vi "S4GUI_002.vi"(7 "Tab ObsEng":enum32{"Obs", "CCD modes", "Eng"}(tab)) -> ()   [LabVIEW 2018] (continued)
          tunnel: w10386 -> [w10388 w10421]
          tunnel: w10385 -> [w10387 w10420]
          tunnel: [w10387 w10398] -> w10384
          tunnel: [w10388 w10399] -> w10383
          frame False {
          }
          frame True {
            # "Carrega a maior temperatura\nentre target atual e o target do controle."
            # "Carrega o valor da temperatura target de acordo com a conf CCD"
            n4383 = call-dynamic "Read AcquisitionD.vi"("error in (no error)"=w10420, "S4ACS_GUI in"=w10421) -> ("error out"=w10424:errorcluster, "Acquisition.lvclass"=w10425:refnum<class "Acquisition.lvclass">, "S4ACS_GUI out"=w10394:refnum<class "S4GUI.lvclass">)  [unwired: 7 in]
            n4384 = call-dynamic "Read Channel.vi"("error in (no error)"=w10424, "Acquisition in"=w10425) -> ("error out"=w10415:errorcluster, "Channel.lvclass"=w10416:refnum<class "Channel.lvclass">, "Acquisition out"=w10395:refnum<class "Acquisition.lvclass">)  [unwired: 7 in]
            n4385 = call-dynamic "ValidateConfig.vi"("error in (no error)"=w10415, "Channel in"=w10416) -> ("error out"=w10409:errorcluster, "Channel out"=w10410:refnum<class "Channel.lvclass">)  [unwired: 7 in, 1 out]
            n4386 = call-dynamic "Read Interface.vi"("error in (no error)"=w10409, "Channel in"=w10410) -> ("error out"=w10413:errorcluster, "Interface.lvclass"=w10414:refnum<class "Interface.lvclass">, "Channel out"=w10418:refnum<class "Channel.lvclass">)  [unwired: 7 in]
            n4387 = call-dynamic "Read Temperature.vi"("error in (no error)"=w10413, "Interface in"=w10414) -> ("error out"=w10412:errorcluster, "Temperature"=w10408:i8, "Interface out"=w10411:refnum<class "Interface.lvclass">)  [unwired: 7 in]
            n4388 = Greater?(x=w10408, y="Target Temp 4") -> (0:w10393:bool)
            n4389 = Select(t=w10408, s=w10393, f="Target Temp 4") -> (s? t:f=w10407:i32)
            n4390 = call-dynamic "Write Temperature.vi"("error in (no error)"=w10412, "Temperature"=w10407, "Interface in"=w10411) -> ("error out"=w10417:errorcluster, "Interface out"=w10419:refnum<class "Interface.lvclass">)  [unwired: 7 in]
            n4391 = call-dynamic "Write Interface.vi"("error in (no error)"=w10417, "Interface.lvclass"=w10419, "Channel in"=w10418) -> ("error out"=w10396:errorcluster, "Channel out"=w10397:refnum<class "Channel.lvclass">)  [unwired: 7 in]
            n4392 = case shown="True" w10393 {
              tunnel: w10396 -> [w10450 w10455]
              tunnel: w10397 -> [w10449 w10457]
              tunnel: [w10448 w10457] -> w10392
              tunnel: [w10447 w10460] -> w10389
              tunnel: w10394 -> [w10427 w10456]
              tunnel: [w10427 w10459] -> w10390
              tunnel: w10395 -> [w10426 w10452]
              tunnel: [w10426 w10458] -> w10391
              frame False {
                n4393 = call-dynamic "Read State Machine.vi"("error in (no error)"=w10450, "Device in"=w10449) -> ("error out"=w10429:errorcluster, "State Machine.lvclass"=w10436:refnum<class "State Machine.lvclass">, "Device out"=w10445:refnum<class "Channel.lvclass">)  [unwired: 7 in]
                n4394 = call-dynamic "Read ref StatesQueue.vi"("error in (no error)"=w10429, "State Machine in"=w10436) -> ("error out"=w10439:errorcluster, "ref StatesQueue"=w10433:refnum<queue>, "State Machine out"=w10435:refnum<class "State Machine.lvclass">)  [unwired: 7 in]
                n4395 = Flush Queue(queue=w10433, error in (no error)=w10439) -> (queue out=w10432:refnum<queue>, error out=w10441:errorcluster)  [unwired: 1 out]
                n4396 = Enqueue Element(queue=w10432, element=u32 35 ("State"), error in (no error)=w10441) -> (queue out=w10431:refnum<queue>, error out=w10442:errorcluster)  [unwired: 1 in, 1 out]
                n4397 = Enqueue Element(queue=w10431, element=u32 37 ("State"), error in (no error)=w10442) -> (queue out=w10430:refnum<queue>, error out=w10440:errorcluster)  [unwired: 1 in, 1 out]
                n4398 = call-dynamic "Write ref StatesQueue.vi"("error in (no error)"=w10440, "ref StatesQueue"=w10430, "State Machine in"=w10435) -> ("error out"=w10428:errorcluster, "State Machine out"=w10434:refnum<class "State Machine.lvclass">)  [unwired: 7 in]
                n4399 = call "Next State.vi"("error in (no error)"=w10428, "New_State"=u32 0, "State Machine in"=w10434) -> ("error out"=w10446:errorcluster, "State Machine out"=w10444:refnum<class "State Machine.lvclass">)  [unwired: 7 in]
                n4400 = call-dynamic "Write State Machine.vi"("error in (no error)"=w10446, "State Machine.lvclass"=w10444, "Device in"=w10445) -> ("error out"=w10447:errorcluster, "Device out"=w10448:refnum<class "Channel.lvclass">)  [unwired: 7 in]
              }
              frame True {
                # "input error"
                n4401 = call-dynamic "Read SET temp error mode.vi"("error in (no error)"=w10455, "S4GUI in"=w10456) -> ("error out"=w10454:errorcluster, "SET temp error mode"=w10451:bool, "S4GUI out"=w10453:refnum<class "S4GUI.lvclass">)  [unwired: 7 in]
                n4402 = case shown="True" w10451 {
                  tunnel: [w10469 w10482] -> w10460
                  tunnel: [w10468 w10490] -> w10459
                  tunnel: [w10464 w10489] -> w10458
                  tunnel: w10454 -> [w10463 w10482]
                  tunnel: w10453 -> [w10461 w10490]
                  tunnel: w10452 -> [w10462 w10489]
                  frame False {
                    # "last error msg"
                    n4403 = call-dynamic "Read sync.vi"("error in (no error)"=w10463, "S4ACS_GUI in"=w10461) -> ("error out"=w10465:errorcluster, "sync"=w10466:bool, "S4ACS_GUI out"=w10467:refnum<class "S4GUI.lvclass">)  [unwired: 7 in]
                    n4404 = case shown="False" w10466 {
                      tunnel: w10465 -> [w10472 w10481]
                      tunnel: [w10471 w10480] -> w10469
                      tunnel: [w10475 w10479] -> w10468
                      tunnel: w10467 -> [w10475 w10477]
                      tunnel: w10462 -> [w10473 w10476]
                      tunnel: [w10470 w10476] -> w10464
                      frame False {
                        n4405 = call-dynamic "Write Acq_state.vi"("error in (no error)"=w10472, "Acq_state"=u32 240, "Acquisition in"=w10473) -> ("error out"=w10471:errorcluster, "Acquisition out"=w10470:refnum<class "Acquisition.lvclass">)  [unwired: 7 in]
                      }
                      frame True {
                        n4406 = call-dynamic "Write Obs_state.vi"("error in (no error)"=w10481, "Obs_state"=u32 240, "S4ACS_GUI in"=w10477) -> ("error out"=w10480:errorcluster, "S4ACS_GUI out"=w10479:refnum<class "S4GUI.lvclass">)  [unwired: 7 in]
                      }
                    }
                  }
                  frame True {
                    w10484 = FALSE ("Wait Until Done")
                    # "popup msg"
                    n4407 = call <vilib>:"Application Directory.vi"() -> ("Application Directory"=w10488:path)
                    n4408 = Build Path(base path=w10488, name or relative path="MsgSetTemp.vi") -> (appended path=w10485:path)
                    n4409 = Open VI Reference(vi path=w10485) -> (vi reference=w10486:refnum<vi>, error out=w10487:errorcluster)  [unwired: 5 in]
                    n4410 = invoke class="VI" method="Run VI"(reference=w10486, error in=w10487, "Wait until done"=w10484, "Auto Dispose Ref"=w10484) -> ()  [unwired: 1 in, 5 out]
                  }
                }
              }
            }
            n4411 = Number To Decimal String(number="Target Temp 4") -> (decimal integer string=w10406:string)  [unwired: 1 in]
            n4412 = call-dynamic "Write Channel.vi"("error in (no error)"=w10389, "Channel.lvclass"=w10392, "Acquisition in"=w10391) -> ("error out"=w10422:errorcluster, "Acquisition out"=w10423:refnum<class "Acquisition.lvclass">)  [unwired: 7 in]
            n4413 = Concatenate Strings("SET TEMP [" ("User Event"), w10406, "] CLICKED - CH4" ("User Event")) -> (w10405:string)
            n4414 = call-dynamic "Write AcquisitionD.vi"("error in (no error)"=w10422, "Acquisition.lvclass"=w10423, "S4ACS_GUI in"=w10390) -> ("error out"=w10400:errorcluster, "S4ACS_GUI out"=w10401:refnum<class "S4GUI.lvclass">)  [unwired: 7 in]
            n4415 = call-dynamic "Write User Event.vi"("error in (no error)"=w10400, "User Event"=w10405, "S4GUI in"=w10401) -> ("error out"=w10398:errorcluster, "S4GUI out"=w10399:refnum<class "S4GUI.lvclass">)  [unwired: 7 in]
          }
        }
      }
      event "SET Temp message": Value Change {
        # "Seleção do modo de apresentação da\nmensagem de erro para o SET de \ntemperatura manual:\nF: via Last Error em vermelho (S4GUI:HandleObservation.vi);\nT: via janela de popup (MsgTempPopup.vi)."
        n4416 = event-data() -> ("NewVal"=w10493:bool)  [unwired: 1 in]
        n4417 = call-dynamic "Write SET temp error mode.vi"("error in (no error)"=w10494, "SET temp error mode"=w10493, "S4GUI in"=w10495) -> ("error out"=w10491:errorcluster, "S4GUI out"=w10492:refnum<class "S4GUI.lvclass">)  [unwired: 7 in]
      }
      event "Avança Estado": Value Change {
        n4418 = event-data() -> ()  [unwired: 1 in, 4 out]
        n4419 = call-dynamic "Read Sync Box.lvclass.vi"("error in (no error)"=w10504, "SPARC4_AC in"=w10505) -> ("error out"=w10517:errorcluster, "Sync Box.lvclass"=w10518:refnum<class "Sync Box.lvclass">, "SPARC4_AC out"=w10509:refnum<class "S4GUI.lvclass">)  [unwired: 7 in]
        n4420 = call-dynamic "Read Trigger.lvclass.vi"("error in (no error)"=w10517, "Sync Box in"=w10518) -> ("error out"=w10515:errorcluster, "Trigger.lvclass"=w10516:refnum<class "Trigger.lvclass">, "Sync Box out"=w10512:refnum<class "Sync Box.lvclass">)  [unwired: 7 in]
        n4421 = call-dynamic "Read State Machine.vi"("error in (no error)"=w10515, "Device in"=w10516) -> ("error out"=w10501:errorcluster, "State Machine.lvclass"=w10502:refnum<class "State Machine.lvclass">, "Device out"=w10513:refnum<class "Trigger.lvclass">)  [unwired: 7 in]
        n4422 = call-dynamic "Read State.vi"("error in (no error)"=w10501, "State Machine in"=w10502) -> ("error out"=w10497:errorcluster, "State"=w10500:i32, "State Machine out"=w10498:refnum<class "State Machine.lvclass">)  [unwired: 7 in]
        n4423 = Increment(x=w10500) -> (x+1=w10499:i32)
        n4424 = call "Next State.vi"("error in (no error)"=w10497, "New_State"=w10499, "State Machine in"=w10498) -> ("error out"=w10511:errorcluster, "State Machine out"=w10514:refnum<class "State Machine.lvclass">)  [unwired: 7 in]
        n4425 = call-dynamic "Write State Machine.vi"("error in (no error)"=w10511, "State Machine.lvclass"=w10514, "Device in"=w10513) -> ("error out"=w10507:errorcluster, "Device out"=w10506:refnum<class "Trigger.lvclass">)  [unwired: 7 in]
        n4426 = call-dynamic "Write Trigger.lvclass.vi"("error in (no error)"=w10507, "Trigger.lvclass"=w10506, "Sync Box in"=w10512) -> ("error out"=w10508:errorcluster, "Sync Box out"=w10510:refnum<class "Sync Box.lvclass">)  [unwired: 7 in]
        n4427 = call-dynamic "Write Sync Box.lvclass.vi"("error in (no error)"=w10508, "Sync Box.lvclass"=w10510, "SPARC4_AC in"=w10509) -> ("error out"=w10503:errorcluster, "SPARC4_AC out"=w10496:refnum<class "S4GUI.lvclass">)  [unwired: 7 in]
      }
      event "DelayA": Value Change {
        n4428 = event-data() -> ("NewVal"=w10520:string)  [unwired: 1 in, 3 out]
        n4429 = call-dynamic "Read Sync Box.lvclass.vi"("error in (no error)"=w10524, "SPARC4_AC in"=w10525) -> ("error out"=w10532:errorcluster, "Sync Box.lvclass"=w10533:refnum<class "Sync Box.lvclass">, "SPARC4_AC out"=w10529:refnum<class "S4GUI.lvclass">)  [unwired: 7 in]
        n4430 = call-dynamic "Read Trigger.lvclass.vi"("error in (no error)"=w10532, "Sync Box in"=w10533) -> ("error out"=w10521:errorcluster, "Trigger.lvclass"=w10522:refnum<class "Trigger.lvclass">, "Sync Box out"=w10531:refnum<class "Sync Box.lvclass">)  [unwired: 7 in]
        n4431 = call-dynamic "Write DelayA.vi"("error in (no error)"=w10521, "DelayA"=w10520, "Trigger in"=w10522) -> ("error out"=w10527:errorcluster, "Trigger out"=w10526:refnum<class "Trigger.lvclass">)  [unwired: 7 in]
        n4432 = call-dynamic "Write Trigger.lvclass.vi"("error in (no error)"=w10527, "Trigger.lvclass"=w10526, "Sync Box in"=w10531) -> ("error out"=w10528:errorcluster, "Sync Box out"=w10530:refnum<class "Sync Box.lvclass">)  [unwired: 7 in]
        n4433 = call-dynamic "Write Sync Box.lvclass.vi"("error in (no error)"=w10528, "Sync Box.lvclass"=w10530, "SPARC4_AC in"=w10529) -> ("error out"=w10523:errorcluster, "SPARC4_AC out"=w10519:refnum<class "S4GUI.lvclass">)  [unwired: 7 in]
      }
      event "DelayB": Value Change {
        n4434 = event-data() -> ("NewVal"=w10535:string)  [unwired: 1 in, 3 out]
        n4435 = call-dynamic "Read Sync Box.lvclass.vi"("error in (no error)"=w10539, "SPARC4_AC in"=w10540) -> ("error out"=w10547:errorcluster, "Sync Box.lvclass"=w10548:refnum<class "Sync Box.lvclass">, "SPARC4_AC out"=w10544:refnum<class "S4GUI.lvclass">)  [unwired: 7 in]
        n4436 = call-dynamic "Read Trigger.lvclass.vi"("error in (no error)"=w10547, "Sync Box in"=w10548) -> ("error out"=w10536:errorcluster, "Trigger.lvclass"=w10537:refnum<class "Trigger.lvclass">, "Sync Box out"=w10546:refnum<class "Sync Box.lvclass">)  [unwired: 7 in]
        n4437 = call-dynamic "Write DelayB.vi"("error in (no error)"=w10536, "DelayB"=w10535, "Trigger in"=w10537) -> ("error out"=w10542:errorcluster, "Trigger out"=w10541:refnum<class "Trigger.lvclass">)  [unwired: 7 in]
        n4438 = call-dynamic "Write Trigger.lvclass.vi"("error in (no error)"=w10542, "Trigger.lvclass"=w10541, "Sync Box in"=w10546) -> ("error out"=w10543:errorcluster, "Sync Box out"=w10545:refnum<class "Sync Box.lvclass">)  [unwired: 7 in]
        n4439 = call-dynamic "Write Sync Box.lvclass.vi"("error in (no error)"=w10543, "Sync Box.lvclass"=w10545, "SPARC4_AC in"=w10544) -> ("error out"=w10538:errorcluster, "SPARC4_AC out"=w10534:refnum<class "S4GUI.lvclass">)  [unwired: 7 in]
      }
      event "DelayC": Value Change {
        n4440 = event-data() -> ("NewVal"=w10550:string)  [unwired: 1 in, 3 out]
        n4441 = call-dynamic "Read Sync Box.lvclass.vi"("error in (no error)"=w10554, "SPARC4_AC in"=w10555) -> ("error out"=w10562:errorcluster, "Sync Box.lvclass"=w10563:refnum<class "Sync Box.lvclass">, "SPARC4_AC out"=w10559:refnum<class "S4GUI.lvclass">)  [unwired: 7 in]
        n4442 = call-dynamic "Read Trigger.lvclass.vi"("error in (no error)"=w10562, "Sync Box in"=w10563) -> ("error out"=w10551:errorcluster, "Trigger.lvclass"=w10552:refnum<class "Trigger.lvclass">, "Sync Box out"=w10561:refnum<class "Sync Box.lvclass">)  [unwired: 7 in]
        n4443 = call-dynamic "Write DelayC.vi"("error in (no error)"=w10551, "DelayC"=w10550, "Trigger in"=w10552) -> ("error out"=w10557:errorcluster, "Trigger out"=w10556:refnum<class "Trigger.lvclass">)  [unwired: 7 in]
        n4444 = call-dynamic "Write Trigger.lvclass.vi"("error in (no error)"=w10557, "Trigger.lvclass"=w10556, "Sync Box in"=w10561) -> ("error out"=w10558:errorcluster, "Sync Box out"=w10560:refnum<class "Sync Box.lvclass">)  [unwired: 7 in]
        n4445 = call-dynamic "Write Sync Box.lvclass.vi"("error in (no error)"=w10558, "Sync Box.lvclass"=w10560, "SPARC4_AC in"=w10559) -> ("error out"=w10553:errorcluster, "SPARC4_AC out"=w10549:refnum<class "S4GUI.lvclass">)  [unwired: 7 in]
      }
      event "DelayD": Value Change {
        n4446 = event-data() -> ("NewVal"=w10565:string)  [unwired: 1 in, 3 out]
        n4447 = call-dynamic "Read Sync Box.lvclass.vi"("error in (no error)"=w10569, "SPARC4_AC in"=w10570) -> ("error out"=w10577:errorcluster, "Sync Box.lvclass"=w10578:refnum<class "Sync Box.lvclass">, "SPARC4_AC out"=w10574:refnum<class "S4GUI.lvclass">)  [unwired: 7 in]
        n4448 = call-dynamic "Read Trigger.lvclass.vi"("error in (no error)"=w10577, "Sync Box in"=w10578) -> ("error out"=w10566:errorcluster, "Trigger.lvclass"=w10567:refnum<class "Trigger.lvclass">, "Sync Box out"=w10576:refnum<class "Sync Box.lvclass">)  [unwired: 7 in]
        n4449 = call-dynamic "Write DelayD.vi"("error in (no error)"=w10566, "DelayD"=w10565, "Trigger in"=w10567) -> ("error out"=w10572:errorcluster, "Trigger out"=w10571:refnum<class "Trigger.lvclass">)  [unwired: 7 in]
        n4450 = call-dynamic "Write Trigger.lvclass.vi"("error in (no error)"=w10572, "Trigger.lvclass"=w10571, "Sync Box in"=w10576) -> ("error out"=w10573:errorcluster, "Sync Box out"=w10575:refnum<class "Sync Box.lvclass">)  [unwired: 7 in]
        n4451 = call-dynamic "Write Sync Box.lvclass.vi"("error in (no error)"=w10573, "Sync Box.lvclass"=w10575, "SPARC4_AC in"=w10574) -> ("error out"=w10568:errorcluster, "SPARC4_AC out"=w10564:refnum<class "S4GUI.lvclass">)  [unwired: 7 in]
      }
      event "WidthA": Value Change {
        n4452 = event-data() -> ("NewVal"=w10580:string)  [unwired: 1 in, 3 out]
        n4453 = call-dynamic "Read Sync Box.lvclass.vi"("error in (no error)"=w10584, "SPARC4_AC in"=w10585) -> ("error out"=w10592:errorcluster, "Sync Box.lvclass"=w10593:refnum<class "Sync Box.lvclass">, "SPARC4_AC out"=w10589:refnum<class "S4GUI.lvclass">)  [unwired: 7 in]
        n4454 = call-dynamic "Read Trigger.lvclass.vi"("error in (no error)"=w10592, "Sync Box in"=w10593) -> ("error out"=w10581:errorcluster, "Trigger.lvclass"=w10582:refnum<class "Trigger.lvclass">, "Sync Box out"=w10591:refnum<class "Sync Box.lvclass">)  [unwired: 7 in]
        n4455 = call-dynamic "Write WidthA.vi"("error in (no error)"=w10581, "WidthA"=w10580, "Trigger in"=w10582) -> ("error out"=w10587:errorcluster, "Trigger out"=w10586:refnum<class "Trigger.lvclass">)  [unwired: 7 in]
        n4456 = call-dynamic "Write Trigger.lvclass.vi"("error in (no error)"=w10587, "Trigger.lvclass"=w10586, "Sync Box in"=w10591) -> ("error out"=w10588:errorcluster, "Sync Box out"=w10590:refnum<class "Sync Box.lvclass">)  [unwired: 7 in]
        n4457 = call-dynamic "Write Sync Box.lvclass.vi"("error in (no error)"=w10588, "Sync Box.lvclass"=w10590, "SPARC4_AC in"=w10589) -> ("error out"=w10583:errorcluster, "SPARC4_AC out"=w10579:refnum<class "S4GUI.lvclass">)  [unwired: 7 in]
      }
      event "WidthB": Value Change {
        n4458 = event-data() -> ("NewVal"=w10595:string)  [unwired: 1 in, 3 out]
        n4459 = call-dynamic "Read Sync Box.lvclass.vi"("error in (no error)"=w10599, "SPARC4_AC in"=w10600) -> ("error out"=w10607:errorcluster, "Sync Box.lvclass"=w10608:refnum<class "Sync Box.lvclass">, "SPARC4_AC out"=w10604:refnum<class "S4GUI.lvclass">)  [unwired: 7 in]
        n4460 = call-dynamic "Read Trigger.lvclass.vi"("error in (no error)"=w10607, "Sync Box in"=w10608) -> ("error out"=w10596:errorcluster, "Trigger.lvclass"=w10597:refnum<class "Trigger.lvclass">, "Sync Box out"=w10606:refnum<class "Sync Box.lvclass">)  [unwired: 7 in]
        n4461 = call-dynamic "Write WidthB.vi"("error in (no error)"=w10596, "WidthB"=w10595, "Trigger in"=w10597) -> ("error out"=w10602:errorcluster, "Trigger out"=w10601:refnum<class "Trigger.lvclass">)  [unwired: 7 in]
        n4462 = call-dynamic "Write Trigger.lvclass.vi"("error in (no error)"=w10602, "Trigger.lvclass"=w10601, "Sync Box in"=w10606) -> ("error out"=w10603:errorcluster, "Sync Box out"=w10605:refnum<class "Sync Box.lvclass">)  [unwired: 7 in]
        n4463 = call-dynamic "Write Sync Box.lvclass.vi"("error in (no error)"=w10603, "Sync Box.lvclass"=w10605, "SPARC4_AC in"=w10604) -> ("error out"=w10598:errorcluster, "SPARC4_AC out"=w10594:refnum<class "S4GUI.lvclass">)  [unwired: 7 in]
      }
      event "WidthC": Value Change {
        n4464 = event-data() -> ("NewVal"=w10610:string)  [unwired: 1 in, 3 out]
        n4465 = call-dynamic "Read Sync Box.lvclass.vi"("error in (no error)"=w10614, "SPARC4_AC in"=w10615) -> ("error out"=w10622:errorcluster, "Sync Box.lvclass"=w10623:refnum<class "Sync Box.lvclass">, "SPARC4_AC out"=w10619:refnum<class "S4GUI.lvclass">)  [unwired: 7 in]
        n4466 = call-dynamic "Read Trigger.lvclass.vi"("error in (no error)"=w10622, "Sync Box in"=w10623) -> ("error out"=w10611:errorcluster, "Trigger.lvclass"=w10612:refnum<class "Trigger.lvclass">, "Sync Box out"=w10621:refnum<class "Sync Box.lvclass">)  [unwired: 7 in]
        n4467 = call-dynamic "Write WidthC.vi"("error in (no error)"=w10611, "WidthC"=w10610, "Trigger in"=w10612) -> ("error out"=w10617:errorcluster, "Trigger out"=w10616:refnum<class "Trigger.lvclass">)  [unwired: 7 in]
        n4468 = call-dynamic "Write Trigger.lvclass.vi"("error in (no error)"=w10617, "Trigger.lvclass"=w10616, "Sync Box in"=w10621) -> ("error out"=w10618:errorcluster, "Sync Box out"=w10620:refnum<class "Sync Box.lvclass">)  [unwired: 7 in]
        n4469 = call-dynamic "Write Sync Box.lvclass.vi"("error in (no error)"=w10618, "Sync Box.lvclass"=w10620, "SPARC4_AC in"=w10619) -> ("error out"=w10613:errorcluster, "SPARC4_AC out"=w10609:refnum<class "S4GUI.lvclass">)  [unwired: 7 in]
      }
      event "WidthD": Value Change {
        n4470 = event-data() -> ("NewVal"=w10625:string)  [unwired: 1 in, 3 out]
        n4471 = call-dynamic "Read Sync Box.lvclass.vi"("error in (no error)"=w10629, "SPARC4_AC in"=w10630) -> ("error out"=w10637:errorcluster, "Sync Box.lvclass"=w10638:refnum<class "Sync Box.lvclass">, "SPARC4_AC out"=w10634:refnum<class "S4GUI.lvclass">)  [unwired: 7 in]
        n4472 = call-dynamic "Read Trigger.lvclass.vi"("error in (no error)"=w10637, "Sync Box in"=w10638) -> ("error out"=w10626:errorcluster, "Trigger.lvclass"=w10627:refnum<class "Trigger.lvclass">, "Sync Box out"=w10636:refnum<class "Sync Box.lvclass">)  [unwired: 7 in]
        n4473 = call-dynamic "Write WidthD.vi"("error in (no error)"=w10626, "WidthD"=w10625, "Trigger in"=w10627) -> ("error out"=w10632:errorcluster, "Trigger out"=w10631:refnum<class "Trigger.lvclass">)  [unwired: 7 in]
        n4474 = call-dynamic "Write Trigger.lvclass.vi"("error in (no error)"=w10632, "Trigger.lvclass"=w10631, "Sync Box in"=w10636) -> ("error out"=w10633:errorcluster, "Sync Box out"=w10635:refnum<class "Sync Box.lvclass">)  [unwired: 7 in]
        n4475 = call-dynamic "Write Sync Box.lvclass.vi"("error in (no error)"=w10633, "Sync Box.lvclass"=w10635, "SPARC4_AC in"=w10634) -> ("error out"=w10628:errorcluster, "SPARC4_AC out"=w10624:refnum<class "S4GUI.lvclass">)  [unwired: 7 in]
      }
      event "WPROT_set": Value Change {
        # "Espera até 10 x 1s = 10s\npara condition de WPROT\n ir para READY"
        n4476 = event-data() -> ()  [unwired: 1 in, 4 out]
        n4477 = call "Read Instrument.lvclass.vi"("error in (no error)"=w10660, "S4ACS_GUI in"=w10661) -> ("error out"=w10658:errorcluster, "Instrument.lvclass"=w10659:refnum<class "Instrument.lvclass">, "S4ACS_GUI out"=w10647:refnum<class "S4GUI.lvclass">)  [unwired: 7 in]
        n4478 = call "Read WPROT.vi"("error in (no error)"=w10658, "Instrument in"=w10659) -> ("error out"=w10654:errorcluster, "Opt_Selector.lvclass"=w10657:refnum<class "Opt_Selector.lvclass">, "Instrument out"=w10650:refnum<class "Instrument.lvclass">)  [unwired: 7 in]
        n4479 = call-dynamic "Read State Machine.vi"("error in (no error)"=w10654, "Device in"=w10657) -> ("error out"=w10653:errorcluster, "State Machine.lvclass"=w10656:refnum<class "State Machine.lvclass">, "Device out"=w10652:refnum<class "Opt_Selector.lvclass">)  [unwired: 7 in]
        n4480 = call "Next State.vi"("error in (no error)"=w10653, "New_State"=1, "State Machine in"=w10656) -> ("error out"=w10641:errorcluster, "State Machine out"=w10643:refnum<class "State Machine.lvclass">)  [unwired: 7 in]
        n4481 = call-dynamic "Write Timer.vi"("error in (no error)"=w10641, "Timer"=u32 10, "State Machine in"=w10643) -> ("error out"=w10640:errorcluster, "State Machine out"=w10642:refnum<class "State Machine.lvclass">)  [unwired: 7 in]
        n4482 = call-dynamic "Write State Machine.vi"("error in (no error)"=w10640, "State Machine.lvclass"=w10642, "Device in"=w10652) -> ("error out"=w10649:errorcluster, "Device out"=w10651:refnum<class "Opt_Selector.lvclass">)  [unwired: 7 in]
        n4483 = call "Write WPROT.vi"("error in (no error)"=w10649, "Opt_Selector.lvclass"=w10651, "Instrument in"=w10650) -> ("error out"=w10646:errorcluster, "Instrument out"=w10648:refnum<class "Instrument.lvclass">)  [unwired: 7 in]
        n4484 = call "Write Instrument.lvclass.vi"("error in (no error)"=w10646, "Instrument.lvclass"=w10648, "S4ACS_GUI in"=w10647) -> ("error out"=w10645:errorcluster, "S4ACS_GUI out"=w10644:refnum<class "S4GUI.lvclass">)  [unwired: 7 in]
      }
      event "TARGET NAME WPROT": Value Change {
        n4485 = event-data() -> ()  [unwired: 1 in, 1 out]
        n4486 = call "Read Instrument.lvclass.vi"("error in (no error)"=w10689, "S4ACS_GUI in"=w10690) -> ("error out"=w10697:errorcluster, "Instrument.lvclass"=w10698:refnum<class "Instrument.lvclass">, "S4ACS_GUI out"=w10692:refnum<class "S4GUI.lvclass">)  [unwired: 7 in]
        n4487 = property on="TARGET NAME WPROT" class="Enum (strict)"() -> ("RingText.Text"=w10688:string)  [unwired: 2 in, 2 out]
        n4488 = Build Array(-1.0 ("element"), 0.0 ("element"), 22.5 ("element"), 45.0 ("element"), 67.5 ("element"), 90.0 ("element"), 112.5 ("element"), 135.0 ("element"), 157.5 ("element"), 180.0 ("element"), 202.5 ("element"), 225.0 ("element"), 247.5 ("element"), 270.0 ("element"), 292.5 ("element"), 315.0 ("element"), 337.5 ("element")) -> (w10680:dbl[])
        n4489 = call "Read WPROT.vi"("error in (no error)"=w10697, "Instrument in"=w10698) -> ("error out"=w10695:errorcluster, "Opt_Selector.lvclass"=w10696:refnum<class "Opt_Selector.lvclass">, "Instrument out"=w10694:refnum<class "Instrument.lvclass">)  [unwired: 7 in]
        n4490 = call "Write target name.vi"("error in (no error)"=w10695, "target name"=w10688, "Optics in"=w10696) -> ("error out"=w10676:errorcluster, "Optics out"=w10677:refnum<class "Opt_Selector.lvclass">)  [unwired: 7 in]
        n4491 = Index Array(array=w10680, index="TARGET NAME WPROT") -> (element=w10678:dbl)
        n4492 = call "Write target.vi"("error in (no error)"=w10676, "target"=w10678, "Optics in"=w10677) -> ("error out"=w10675:errorcluster, "Optics out"=w10674:refnum<class "Opt_Selector.lvclass">)  [unwired: 7 in]
        n4493 = call "Write WPROT.vi"("error in (no error)"=w10675, "Opt_Selector.lvclass"=w10674, "Instrument in"=w10694) -> ("error out"=w10691:errorcluster, "Instrument out"=w10693:refnum<class "Instrument.lvclass">)  [unwired: 7 in]
        n4494 = call "Write Instrument.lvclass.vi"("error in (no error)"=w10691, "Instrument.lvclass"=w10693, "S4ACS_GUI in"=w10692) -> ("error out"=w10687:errorcluster, "S4ACS_GUI out"=w10662:refnum<class "S4GUI.lvclass">)  [unwired: 7 in]
      }
      event "TARGET NAME WPSEL": Value Change {
        n4495 = event-data() -> ()  [unwired: 1 in, 1 out]
        n4496 = call "Read Instrument.lvclass.vi"("error in (no error)"=w10713, "S4ACS_GUI in"=w10714) -> ("error out"=w10721:errorcluster, "Instrument.lvclass"=w10722:refnum<class "Instrument.lvclass">, "S4ACS_GUI out"=w10716:refnum<class "S4GUI.lvclass">)  [unwired: 7 in]
        n4497 = property on="TARGET NAME WPSEL" class="Enum (strict)"() -> ("RingText.Text"=w10700:string)  [unwired: 2 in, 2 out]
        n4498 = Build Array(-1.0 ("element"), 80.0 ("element"), 0.0 ("element"), 160.0 ("element")) -> (w10707:dbl[])
        n4499 = call "Read WPSEL.vi"("error in (no error)"=w10721, "Instrument in"=w10722) -> ("error out"=w10719:errorcluster, "Opt_Selector.lvclass"=w10720:refnum<class "Opt_Selector.lvclass">, "Instrument out"=w10718:refnum<class "Instrument.lvclass">)  [unwired: 7 in]
        n4500 = call "Write target name.vi"("error in (no error)"=w10719, "target name"=w10700, "Optics in"=w10720) -> ("error out"=w10704:errorcluster, "Optics out"=w10705:refnum<class "Opt_Selector.lvclass">)  [unwired: 7 in]
        n4501 = Index Array(array=w10707, index="TARGET NAME WPSEL") -> (element=w10706:dbl)
        n4502 = call "Write target.vi"("error in (no error)"=w10704, "target"=w10706, "Optics in"=w10705) -> ("error out"=w10703:errorcluster, "Optics out"=w10702:refnum<class "Opt_Selector.lvclass">)  [unwired: 7 in]
        n4503 = call "Write WPSEL.vi"("error in (no error)"=w10703, "Opt_Selector.lvclass"=w10702, "Instrument in"=w10718) -> ("error out"=w10715:errorcluster, "Instrument out"=w10717:refnum<class "Instrument.lvclass">)  [unwired: 7 in]
        n4504 = call "Write Instrument.lvclass.vi"("error in (no error)"=w10715, "Instrument.lvclass"=w10717, "S4ACS_GUI in"=w10716) -> ("error out"=w10712:errorcluster, "S4ACS_GUI out"=w10699:refnum<class "S4GUI.lvclass">)  [unwired: 7 in]
      }
      event "Lambda Selector": Value Change {
        n4505 = event-data() -> ("NewVal"=w10724:u16)  [unwired: 1 in, 1 out]
        n4506 = call "Read Instrument.lvclass.vi"("error in (no error)"=w10755, "S4ACS_GUI in"=w10756) -> ("error out"=w10757:errorcluster, "Instrument.lvclass"=w10732:refnum<class "Instrument.lvclass">, "S4ACS_GUI out"=w10729:refnum<class "S4GUI.lvclass">)  [unwired: 7 in]
        n4507 = Build Array(80.0 ("element"), 0.0 ("element"), 160.0 ("element")) -> (w10750:dbl[])
        n4508 = property on="Lambda Selector" class="Ring (strict)"() -> ("RingText.Text"=w10730:string)  [unwired: 2 in, 2 out]
        n4509 = call "Read WPSEL.vi"("error in (no error)"=w10757, "Instrument in"=w10732) -> ("error out"=w10739:errorcluster, "Opt_Selector.lvclass"=w10738:refnum<class "Opt_Selector.lvclass">, "Instrument out"=w10731:refnum<class "Instrument.lvclass">)  [unwired: 7 in]
        n4510 = Index Array(array=w10750, index=w10724) -> (element=w10749:dbl)
        n4511 = call "Write target.vi"("error in (no error)"=w10739, "target"=w10749, "Optics in"=w10738) -> ("error out"=w10736:errorcluster, "Optics out"=w10737:refnum<class "Opt_Selector.lvclass">)  [unwired: 7 in]
        n4512 = case shown="\"Lambda/4\"" w10730 {
          selector: w10730 -> [w10760 _ _]
          tunnel: [w10760 "ON" "ON"] -> w10741
          tunnel: [0.0 ("element") 30.0 ("element") 30.0 ("element")] -> w10740
          tunnel: [w10760 "L/2" "L/4"] -> w10733
          frame "OFF", Default {
            n4513 = property on="Calibrator Selector" class="Ring (strict)"("DisabledEnum"=T12."Disabled and Grayed Out" ("Disabled")) -> ()  [unwired: 2 in, 2 out]
          }
          frame "Lambda/2" {
            n4514 = property on="Calibrator Selector" class="Ring (strict)"("DisabledEnum"=T12."Enabled" ("Disabled")) -> ()  [unwired: 2 in, 2 out]
          }
          frame "Lambda/4" {
            n4515 = property on="Calibrator Selector" class="Ring (strict)"("DisabledEnum"=T12."Enabled" ("Disabled")) -> ()  [unwired: 2 in, 2 out]
          }
        }
        n4516 = call "Write target name.vi"("error in (no error)"=w10736, "target name"=w10733, "Optics in"=w10737) -> ("error out"=w10735:errorcluster, "Optics out"=w10734:refnum<class "Opt_Selector.lvclass">)  [unwired: 7 in]
        n4517 = call "Write WPSEL.vi"("error in (no error)"=w10735, "Opt_Selector.lvclass"=w10734, "Instrument in"=w10731) -> ("error out"=w10726:errorcluster, "Instrument out"=w10725:refnum<class "Instrument.lvclass">)  [unwired: 7 in]
        n4518 = call "Read ASEL.vi"("error in (no error)"=w10726, "Instrument in"=w10725) -> ("error out"=w10746:errorcluster, "Opt_Selector.lvclass"=w10744:refnum<class "Opt_Selector.lvclass">, "Instrument out"=w10728:refnum<class "Instrument.lvclass">)  [unwired: 7 in]
        n4519 = call "Write target name.vi"("error in (no error)"=w10746, "target name"=w10741, "Optics in"=w10744) -> ("error out"=w10747:errorcluster, "Optics out"=w10743:refnum<class "Opt_Selector.lvclass">)  [unwired: 7 in]
        n4520 = call "Write target.vi"("error in (no error)"=w10747, "target"=w10740, "Optics in"=w10743) -> ("error out"=w10748:errorcluster, "Optics out"=w10742:refnum<class "Opt_Selector.lvclass">)  [unwired: 7 in]
        n4521 = call "Write ASEL.vi"("error in (no error)"=w10748, "Opt_Selector.lvclass"=w10742, "Instrument in"=w10728) -> ("error out"=w10745:errorcluster, "Instrument out"=w10727:refnum<class "Instrument.lvclass">)  [unwired: 7 in]
        n4522 = call "Write Instrument.lvclass.vi"("error in (no error)"=w10745, "Instrument.lvclass"=w10727, "S4ACS_GUI in"=w10729) -> ("error out"=w10754:errorcluster, "S4ACS_GUI out"=w10723:refnum<class "S4GUI.lvclass">)  [unwired: 7 in]
      }
      event "Calibrator Selector": Value Change {
        n4523 = event-data() -> ()  [unwired: 1 in, 6 out]
        n4524 = call "Read Instrument.lvclass.vi"("error in (no error)"=w10789, "S4ACS_GUI in"=w10790) -> ("error out"=w10793:errorcluster, "Instrument.lvclass"=w10794:refnum<class "Instrument.lvclass">, "S4ACS_GUI out"=w10791:refnum<class "S4GUI.lvclass">)  [unwired: 7 in]
        n4525 = Build Array(0.0 ("element"), 72.0 ("element"), 144.0 ("element"), 216.0 ("element"), 288.0 ("element")) -> (w10784:dbl[])
        n4526 = call "Read CALW.vi"("error in (no error)"=w10793, "Instrument in"=w10794) -> ("error out"=w10782:errorcluster, "Opt_Selector.lvclass"=w10781:refnum<class "Opt_Selector.lvclass">, "Instrument out"=w10792:refnum<class "Instrument.lvclass">)  [unwired: 7 in]
        n4527 = Index Array(array=w10784, index="Calibrator Selector") -> (element=w10783:dbl)
        n4528 = call "Write target.vi"("error in (no error)"=w10782, "target"=w10783, "Optics in"=w10781) -> ("error out"=w10779:errorcluster, "Optics out"=w10780:refnum<class "Opt_Selector.lvclass">)  [unwired: 7 in]
        n4529 = property on="Calibrator Selector" class="Ring (strict)"() -> ("RingText.Text"=w10775:string)  [unwired: 2 in, 2 out]
        n4530 = case shown="\"POLARIZER\"" w10775 {
          selector: w10775 -> [_ w10796 w10797 w10798 w10799]
          tunnel: ["OFF" w10796 w10797 w10798 w10799] -> w10776
          frame "OFF", Default {
          }
          frame "POLARIZER" {
          }
          frame "DEPOLARIZER" {
          }
          frame "PINHOLE" {
          }
          frame "SHUTTER" {
          }
        }
        n4531 = call "Write target name.vi"("error in (no error)"=w10779, "target name"=w10776, "Optics in"=w10780) -> ("error out"=w10778:errorcluster, "Optics out"=w10777:refnum<class "Opt_Selector.lvclass">)  [unwired: 7 in]
        n4532 = call "Write CALW.vi"("error in (no error)"=w10778, "Opt_Selector.lvclass"=w10777, "Instrument in"=w10792) -> ("error out"=w10772:errorcluster, "Instrument out"=w10773:refnum<class "Instrument.lvclass">)  [unwired: 7 in]
        n4533 = call "Write Instrument.lvclass.vi"("error in (no error)"=w10772, "Instrument.lvclass"=w10773, "S4ACS_GUI in"=w10791) -> ("error out"=w10788:errorcluster, "S4ACS_GUI out"=w10771:refnum<class "S4GUI.lvclass">)  [unwired: 7 in]
      }
      event "TARGET NAME CALW": Value Change {
        # "aqui também"
        # "OV20230825: Valores da sequência original"
        n4534 = event-data() -> ()  [unwired: 1 in, 6 out]
        n4535 = call "Read Instrument.lvclass.vi"("error in (no error)"=w10816, "S4ACS_GUI in"=w10817) -> ("error out"=w10824:errorcluster, "Instrument.lvclass"=w10825:refnum<class "Instrument.lvclass">, "S4ACS_GUI out"=w10819:refnum<class "S4GUI.lvclass">)  [unwired: 7 in]
        n4536 = property on="TARGET NAME CALW" class="Enum (strict)"() -> ("RingText.Text"=w10800:string)  [unwired: 2 in, 2 out]
        n4537 = Build Array(-1.0 ("element"), 0.0 ("element"), 72.0 ("element"), 144.0 ("element"), 216.0 ("element"), 288.0 ("element")) -> (w10810:dbl[])
        n4538 = call "Read CALW.vi"("error in (no error)"=w10824, "Instrument in"=w10825) -> ("error out"=w10822:errorcluster, "Opt_Selector.lvclass"=w10823:refnum<class "Opt_Selector.lvclass">, "Instrument out"=w10821:refnum<class "Instrument.lvclass">)  [unwired: 7 in]
        n4539 = call "Write target name.vi"("error in (no error)"=w10822, "target name"=w10800, "Optics in"=w10823) -> ("error out"=w10807:errorcluster, "Optics out"=w10808:refnum<class "Opt_Selector.lvclass">)  [unwired: 7 in]
        n4540 = Index Array(array=w10810, index="TARGET NAME CALW") -> (element=w10809:dbl)
        n4541 = call "Write target.vi"("error in (no error)"=w10807, "target"=w10809, "Optics in"=w10808) -> ("error out"=w10806:errorcluster, "Optics out"=w10805:refnum<class "Opt_Selector.lvclass">)  [unwired: 7 in]
        n4542 = call "Write CALW.vi"("error in (no error)"=w10806, "Opt_Selector.lvclass"=w10805, "Instrument in"=w10821) -> ("error out"=w10818:errorcluster, "Instrument out"=w10820:refnum<class "Instrument.lvclass">)  [unwired: 7 in]
        n4543 = call "Write Instrument.lvclass.vi"("error in (no error)"=w10818, "Instrument.lvclass"=w10820, "S4ACS_GUI in"=w10819) -> ("error out"=w10815:errorcluster, "S4ACS_GUI out"=w10801:refnum<class "S4GUI.lvclass">)  [unwired: 7 in]
      }
      event "TARGET NAME ASEL": Value Change {
        n4544 = event-data() -> ()  [unwired: 1 in, 6 out]
        n4545 = call "Read Instrument.lvclass.vi"("error in (no error)"=w10839, "S4ACS_GUI in"=w10840) -> ("error out"=w10847:errorcluster, "Instrument.lvclass"=w10848:refnum<class "Instrument.lvclass">, "S4ACS_GUI out"=w10842:refnum<class "S4GUI.lvclass">)  [unwired: 7 in]
        n4546 = Build Array(-1.0 ("element"), 0.0 ("element"), 30.0 ("element")) -> (w10834:dbl[])
        n4547 = call "Read ASEL.vi"("error in (no error)"=w10847, "Instrument in"=w10848) -> ("error out"=w10845:errorcluster, "Opt_Selector.lvclass"=w10846:refnum<class "Opt_Selector.lvclass">, "Instrument out"=w10844:refnum<class "Instrument.lvclass">)  [unwired: 7 in]
        n4548 = property on="TARGET NAME ASEL" class="Enum (strict)"() -> ("RingText.Text"=w10828:string)  [unwired: 2 in, 2 out]
        n4549 = call "Write target name.vi"("error in (no error)"=w10845, "target name"=w10828, "Optics in"=w10846) -> ("error out"=w10831:errorcluster, "Optics out"=w10832:refnum<class "Opt_Selector.lvclass">)  [unwired: 7 in]
        n4550 = Index Array(array=w10834, index="TARGET NAME ASEL") -> (element=w10833:dbl)
        n4551 = call "Write target.vi"("error in (no error)"=w10831, "target"=w10833, "Optics in"=w10832) -> ("error out"=w10830:errorcluster, "Optics out"=w10829:refnum<class "Opt_Selector.lvclass">)  [unwired: 7 in]
        n4552 = call "Write ASEL.vi"("error in (no error)"=w10830, "Opt_Selector.lvclass"=w10829, "Instrument in"=w10844) -> ("error out"=w10841:errorcluster, "Instrument out"=w10843:refnum<class "Instrument.lvclass">)  [unwired: 7 in]
        n4553 = call "Write Instrument.lvclass.vi"("error in (no error)"=w10841, "Instrument.lvclass"=w10843, "S4ACS_GUI in"=w10842) -> ("error out"=w10838:errorcluster, "S4ACS_GUI out"=w10826:refnum<class "S4GUI.lvclass">)  [unwired: 7 in]
      }
      event "WPROT_stop": Value Change {
        n4554 = event-data() -> ()  [unwired: 1 in, 4 out]
        n4555 = call "Read Instrument.lvclass.vi"("error in (no error)"=w10867, "S4ACS_GUI in"=w10868) -> ("error out"=w10865:errorcluster, "Instrument.lvclass"=w10866:refnum<class "Instrument.lvclass">, "S4ACS_GUI out"=w10852:refnum<class "S4GUI.lvclass">)  [unwired: 7 in]
        n4556 = call "Read WPROT.vi"("error in (no error)"=w10865, "Instrument in"=w10866) -> ("error out"=w10861:errorcluster, "Opt_Selector.lvclass"=w10864:refnum<class "Opt_Selector.lvclass">, "Instrument out"=w10855:refnum<class "Instrument.lvclass">)  [unwired: 7 in]
        n4557 = call-dynamic "Read State Machine.vi"("error in (no error)"=w10861, "Device in"=w10864) -> ("error out"=w10860:errorcluster, "State Machine.lvclass"=w10863:refnum<class "State Machine.lvclass">, "Device out"=w10857:refnum<class "Opt_Selector.lvclass">)  [unwired: 7 in]
        n4558 = call "Next State.vi"("error in (no error)"=w10860, "New_State"=10, "State Machine in"=w10863) -> ("error out"=w10859:errorcluster, "State Machine out"=w10858:refnum<class "State Machine.lvclass">)  [unwired: 7 in]
        n4559 = call-dynamic "Write State Machine.vi"("error in (no error)"=w10859, "State Machine.lvclass"=w10858, "Device in"=w10857) -> ("error out"=w10854:errorcluster, "Device out"=w10856:refnum<class "Opt_Selector.lvclass">)  [unwired: 7 in]
        n4560 = call "Write WPROT.vi"("error in (no error)"=w10854, "Opt_Selector.lvclass"=w10856, "Instrument in"=w10855) -> ("error out"=w10851:errorcluster, "Instrument out"=w10853:refnum<class "Instrument.lvclass">)  [unwired: 7 in]
        n4561 = call "Write Instrument.lvclass.vi"("error in (no error)"=w10851, "Instrument.lvclass"=w10853, "S4ACS_GUI in"=w10852) -> ("error out"=w10850:errorcluster, "S4ACS_GUI out"=w10849:refnum<class "S4GUI.lvclass">)  [unwired: 7 in]
      }
      event "WPROT_init": Value Change {
        n4562 = event-data() -> ()  [unwired: 1 in, 4 out]
        n4563 = call "Read Instrument.lvclass.vi"("error in (no error)"=w10887, "S4ACS_GUI in"=w10888) -> ("error out"=w10885:errorcluster, "Instrument.lvclass"=w10886:refnum<class "Instrument.lvclass">, "S4ACS_GUI out"=w10872:refnum<class "S4GUI.lvclass">)  [unwired: 7 in]
        n4564 = call "Read WPROT.vi"("error in (no error)"=w10885, "Instrument in"=w10886) -> ("error out"=w10881:errorcluster, "Opt_Selector.lvclass"=w10884:refnum<class "Opt_Selector.lvclass">, "Instrument out"=w10875:refnum<class "Instrument.lvclass">)  [unwired: 7 in]
        n4565 = call-dynamic "Read State Machine.vi"("error in (no error)"=w10881, "Device in"=w10884) -> ("error out"=w10880:errorcluster, "State Machine.lvclass"=w10883:refnum<class "State Machine.lvclass">, "Device out"=w10877:refnum<class "Opt_Selector.lvclass">)  [unwired: 7 in]
        n4566 = call "Next State.vi"("error in (no error)"=w10880, "New_State"=30, "State Machine in"=w10883) -> ("error out"=w10879:errorcluster, "State Machine out"=w10878:refnum<class "State Machine.lvclass">)  [unwired: 7 in]
        n4567 = call-dynamic "Write State Machine.vi"("error in (no error)"=w10879, "State Machine.lvclass"=w10878, "Device in"=w10877) -> ("error out"=w10874:errorcluster, "Device out"=w10876:refnum<class "Opt_Selector.lvclass">)  [unwired: 7 in]
        n4568 = call "Write WPROT.vi"("error in (no error)"=w10874, "Opt_Selector.lvclass"=w10876, "Instrument in"=w10875) -> ("error out"=w10871:errorcluster, "Instrument out"=w10873:refnum<class "Instrument.lvclass">)  [unwired: 7 in]
        n4569 = call "Write Instrument.lvclass.vi"("error in (no error)"=w10871, "Instrument.lvclass"=w10873, "S4ACS_GUI in"=w10872) -> ("error out"=w10870:errorcluster, "S4ACS_GUI out"=w10869:refnum<class "S4GUI.lvclass">)  [unwired: 7 in]
      }
      event "WPSEL_target": Value Change {
        n4570 = event-data() -> ("NewVal"=w10898:dbl)  [unwired: 1 in, 3 out]
        n4571 = call "Read Instrument.lvclass.vi"("error in (no error)"=w10902, "S4ACS_GUI in"=w10903) -> ("error out"=w10900:errorcluster, "Instrument.lvclass"=w10901:refnum<class "Instrument.lvclass">, "S4ACS_GUI out"=w10892:refnum<class "S4GUI.lvclass">)  [unwired: 7 in]
        n4572 = call "Read WPSEL.vi"("error in (no error)"=w10900, "Instrument in"=w10901) -> ("error out"=w10897:errorcluster, "Opt_Selector.lvclass"=w10899:refnum<class "Opt_Selector.lvclass">, "Instrument out"=w10895:refnum<class "Instrument.lvclass">)  [unwired: 7 in]
        n4573 = call "Write target.vi"("error in (no error)"=w10897, "target"=w10898, "Optics in"=w10899) -> ("error out"=w10894:errorcluster, "Optics out"=w10896:refnum<class "Opt_Selector.lvclass">)  [unwired: 7 in]
        n4574 = call "Write WPSEL.vi"("error in (no error)"=w10894, "Opt_Selector.lvclass"=w10896, "Instrument in"=w10895) -> ("error out"=w10891:errorcluster, "Instrument out"=w10893:refnum<class "Instrument.lvclass">)  [unwired: 7 in]
        n4575 = call "Write Instrument.lvclass.vi"("error in (no error)"=w10891, "Instrument.lvclass"=w10893, "S4ACS_GUI in"=w10892) -> ("error out"=w10890:errorcluster, "S4ACS_GUI out"=w10889:refnum<class "S4GUI.lvclass">)  [unwired: 7 in]
      }
      event "WPSEL_set": Value Change {
        n4576 = event-data() -> ()  [unwired: 1 in, 4 out]
        n4577 = call "Read Instrument.lvclass.vi"("error in (no error)"=w10922, "S4ACS_GUI in"=w10923) -> ("error out"=w10920:errorcluster, "Instrument.lvclass"=w10921:refnum<class "Instrument.lvclass">, "S4ACS_GUI out"=w10908:refnum<class "S4GUI.lvclass">)  [unwired: 7 in]
        n4578 = call "Read WPSEL.vi"("error in (no error)"=w10920, "Instrument in"=w10921) -> ("error out"=w10917:errorcluster, "Opt_Selector.lvclass"=w10919:refnum<class "Opt_Selector.lvclass">, "Instrument out"=w10911:refnum<class "Instrument.lvclass">)  [unwired: 7 in]
        n4579 = call-dynamic "Read State Machine.vi"("error in (no error)"=w10917, "Device in"=w10919) -> ("error out"=w10916:errorcluster, "State Machine.lvclass"=w10905:refnum<class "State Machine.lvclass">, "Device out"=w10913:refnum<class "Opt_Selector.lvclass">)  [unwired: 7 in]
        n4580 = call "Next State.vi"("error in (no error)"=w10916, "New_State"=1, "State Machine in"=w10905) -> ("error out"=w10915:errorcluster, "State Machine out"=w10914:refnum<class "State Machine.lvclass">)  [unwired: 7 in]
        n4581 = call-dynamic "Write State Machine.vi"("error in (no error)"=w10915, "State Machine.lvclass"=w10914, "Device in"=w10913) -> ("error out"=w10910:errorcluster, "Device out"=w10912:refnum<class "Opt_Selector.lvclass">)  [unwired: 7 in]
        n4582 = call "Write WPSEL.vi"("error in (no error)"=w10910, "Opt_Selector.lvclass"=w10912, "Instrument in"=w10911) -> ("error out"=w10907:errorcluster, "Instrument out"=w10909:refnum<class "Instrument.lvclass">)  [unwired: 7 in]
        n4583 = call "Write Instrument.lvclass.vi"("error in (no error)"=w10907, "Instrument.lvclass"=w10909, "S4ACS_GUI in"=w10908) -> ("error out"=w10906:errorcluster, "S4ACS_GUI out"=w10904:refnum<class "S4GUI.lvclass">)  [unwired: 7 in]
      }
      event "Set Waveplate": Value Change {
        # "OV20230825: Sequência de\nvalores originais."
        # "Garantir que, quando em POLARIMETRIA, pelo menos WP1 esteja selecionado."
        n4584 = event-data() -> ()  [unwired: 1 in, 4 out]
        n4585 = local read "Lambda Selector"() -> (w11027:u16)
        n4586 = property on="Calibrator Selector" class="Ring (strict)"() -> ("RingText.Text"=w11008:string)  [unwired: 2 in, 2 out]
        n4587 = call "Read Instrument.lvclass.vi"("error in (no error)"=w11007, "S4ACS_GUI in"=w11006) -> ("error out"=w11025:errorcluster, "Instrument.lvclass"=w11026:refnum<class "Instrument.lvclass">, "S4ACS_GUI out"=w11023:refnum<class "S4GUI.lvclass">)  [unwired: 7 in]
        n4588 = Build Array(0.0 ("element"), 72.0 ("element"), 144.0 ("element"), 216.0 ("element"), 288.0 ("element")) -> (w11019:dbl[])
        n4589 = local read "Calibrator Selector"() -> (w11009:u16)
        n4590 = Build Array(80.0 ("element"), 0.0 ("element"), 160.0 ("element")) -> (w11053:dbl[])
        n4591 = property on="Lambda Selector" class="Ring (strict)"() -> ("RingText.Text"=w11028:string)  [unwired: 2 in, 2 out]
        n4592 = call "Read CALW.vi"("error in (no error)"=w11025, "Instrument in"=w11026) -> ("error out"=w11017:errorcluster, "Opt_Selector.lvclass"=w11016:refnum<class "Opt_Selector.lvclass">, "Instrument out"=w11024:refnum<class "Instrument.lvclass">)  [unwired: 7 in]
        n4593 = Index Array(array=w11019, index=w11009) -> (element=w11018:dbl)
        n4594 = Index Array(array=w11053, index=w11027) -> (element=w11052:dbl)
        n4595 = call "Write target.vi"("error in (no error)"=w11017, "target"=w11018, "Optics in"=w11016) -> ("error out"=w11014:errorcluster, "Optics out"=w11015:refnum<class "Opt_Selector.lvclass">)  [unwired: 7 in]
        n4596 = case shown="\"OFF\", Default" w11008 {
          tunnel: ["OFF" w11282 "PINHOLE" "SHUTTER" w11287] -> w10926
          frame "OFF", Default {
          }
          frame "POLARIZER" {
            n4597 = disable-structure shown="Enabled" {
              disable-tunnel: ["POLARIZER" "DEPOLARIZER"] -> w11282
              frame Enabled {
              }
              frame Disabled {
                # "OV20230426: Montagem do CALW\nestá com POL e DEPOL invertidos"
              }
            }
          }
          frame "PINHOLE" {
          }
          frame "SHUTTER" {
          }
          frame "DEPOLARIZER" {
            n4598 = disable-structure shown="Enabled" {
              disable-tunnel: ["POLARIZER" "DEPOLARIZER"] -> w11287
              frame Disabled {
                # "OV20230426: Montagem do CALW\nestá com POL e DEPOL invertidos"
              }
              frame Enabled {
              }
            }
          }
        }
        n4599 = case shown="\"OFF\", Default" w11028 {
          tunnel: [w11290 "ON" "ON"] -> w10939
          tunnel: [w11291 w11292 w11295] -> w11044
          tunnel: [w11290 "L/2" "L/4"] -> w10924
          tunnel: [w11291 w11292 w11295] -> w10928
          frame "OFF", Default {
            w11290 = "OFF"
            w11291 = 0.0 ("element")
            n4600 = property on="Lambda Selector" class="Ring (strict)"("RingText.Text"=w11290) -> ()  [unwired: 2 in, 2 out]
          }
          frame "Lambda/2" {
            w11292 = 30.0 ("element")
          }
          frame "Lambda/4" {
            w11295 = 30.0 ("element")
          }
        }
        n4601 = call "Write target name.vi"("error in (no error)"=w11014, "target name"=w10926, "Optics in"=w11015) -> ("error out"=w11013:errorcluster, "Optics out"=w11012:refnum<class "Opt_Selector.lvclass">)  [unwired: 7 in]
        n4602 = call "Write CALW.vi"("error in (no error)"=w11013, "Opt_Selector.lvclass"=w11012, "Instrument in"=w11024) -> ("error out"=w11010:errorcluster, "Instrument out"=w11011:refnum<class "Instrument.lvclass">)  [unwired: 7 in]
        n4603 = Equal To 0?(x=w10928) -> (x = 0?=w10929:bool)
        n4604 = call "Write Instrument.lvclass.vi"("error in (no error)"=w11010, "Instrument.lvclass"=w11011, "S4ACS_GUI in"=w11023) -> ("error out"=w11004:errorcluster, "S4ACS_GUI out"=w11005:refnum<class "S4GUI.lvclass">)  [unwired: 7 in]
        n4605 = call "Read Instrument.lvclass.vi"("error in (no error)"=w11004, "S4ACS_GUI in"=w11005) -> ("error out"=w11057:errorcluster, "Instrument.lvclass"=w11037:refnum<class "Instrument.lvclass">, "S4ACS_GUI out"=w11035:refnum<class "S4GUI.lvclass">)  [unwired: 7 in]
        n4606 = call "Read WPSEL.vi"("error in (no error)"=w11057, "Instrument in"=w11037) -> ("error out"=w11043:errorcluster, "Opt_Selector.lvclass"=w11042:refnum<class "Opt_Selector.lvclass">, "Instrument out"=w11036:refnum<class "Instrument.lvclass">)  [unwired: 7 in]
        n4607 = call "Write target.vi"("error in (no error)"=w11043, "target"=w11052, "Optics in"=w11042) -> ("error out"=w11040:errorcluster, "Optics out"=w11041:refnum<class "Opt_Selector.lvclass">)  [unwired: 7 in]
        n4608 = call "Write target name.vi"("error in (no error)"=w11040, "target name"=w10924, "Optics in"=w11041) -> ("error out"=w11039:errorcluster, "Optics out"=w11038:refnum<class "Opt_Selector.lvclass">)  [unwired: 7 in]
        n4609 = call "Write WPSEL.vi"("error in (no error)"=w11039, "Opt_Selector.lvclass"=w11038, "Instrument in"=w11036) -> ("error out"=w11032:errorcluster, "Instrument out"=w11031:refnum<class "Instrument.lvclass">)  [unwired: 7 in]
        n4610 = call "Read ASEL.vi"("error in (no error)"=w11032, "Instrument in"=w11031) -> ("error out"=w11049:errorcluster, "Opt_Selector.lvclass"=w11047:refnum<class "Opt_Selector.lvclass">, "Instrument out"=w11034:refnum<class "Instrument.lvclass">)  [unwired: 7 in]
        n4611 = call "Write target name.vi"("error in (no error)"=w11049, "target name"=w10939, "Optics in"=w11047) -> ("error out"=w11050:errorcluster, "Optics out"=w11046:refnum<class "Opt_Selector.lvclass">)  [unwired: 7 in]
        n4612 = Select(t="OFF", s=w10929, f=w10926) -> (s? t:f=w10927:string)
        n4613 = call "Write target.vi"("error in (no error)"=w11050, "target"=w11044, "Optics in"=w11046) -> ("error out"=w11051:errorcluster, "Optics out"=w11045:refnum<class "Opt_Selector.lvclass">)  [unwired: 7 in]
        n4614 = call "Write ASEL.vi"("error in (no error)"=w11051, "Opt_Selector.lvclass"=w11045, "Instrument in"=w11034) -> ("error out"=w11048:errorcluster, "Instrument out"=w11033:refnum<class "Instrument.lvclass">)  [unwired: 7 in]
